vi "Add to Scene.vi"(8 "error in (no error)":errorcluster, 9 "Color":T1={"Red"=0.0, "Green"=0.0, "Blue"=1.0, "Alpha"=1.0}, 10 "Scene Object In":refnum<vi>, 11 "Cube in":refnum<class "Cube.lvclass">) -> (0 "error out":errorcluster, 2 "Scene Object Out":refnum<vi>, 3 "Cube out":refnum<class "Cube.lvclass">)   [LabVIEW 2019, in "22.lvlib" / "Cube.lvclass"]
uses:
  Cube.lvclass
  <vilib>/picture/3D Picture Control/Object/Create Object (drawable).vi
  <vilib>/picture/3D Picture Control/Object/Create Object (name).vi
  <vilib>/picture/3D Picture Control/Object/Add Object (no reference).vi
  <vilib>/picture/3D Picture Control/Object/Add Object (reference).vi
  <vilib>/picture/3D Picture Control/NI_3D Picture Control.lvlib
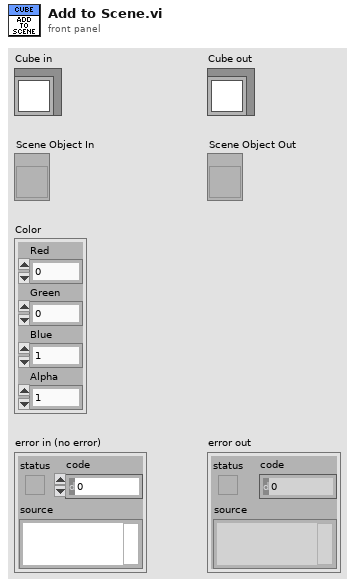
[diagram p1: front panel]
types:
  T1 = cluster{"Red":sgl, "Green":sgl, "Blue":sgl, "Alpha":sgl}
  T2 = cluster{"xmin":i64, "xmax":i64, "ymin":i64, "ymax":i64, "zmin":i64, "zmax":i64}
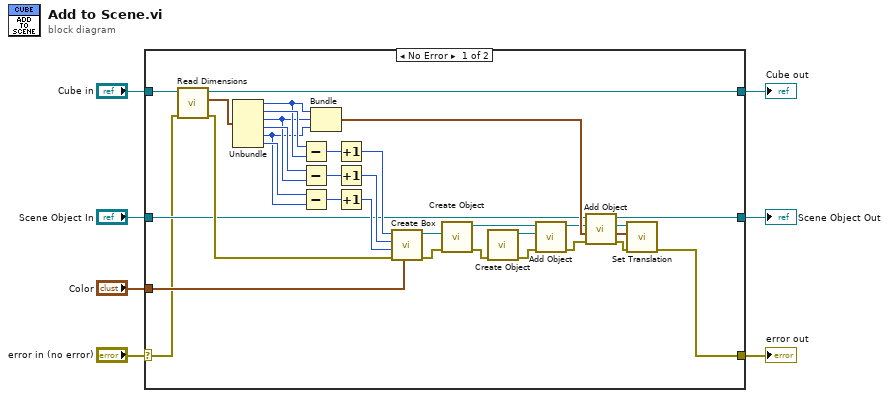
[diagram p0: block diagram]
diagram:
  n1 = case shown="No Error" "error in (no error)" {
    selector: "error in (no error)" -> [w9 w42]
    tunnel: [w13 w42] -> w6
    tunnel: [w39 w41] -> w4
    tunnel: "Cube in" -> [w38 w41]
    tunnel: "Color" -> [w17 _]
    tunnel: "Scene Object In" -> [w15 w40]
    tunnel: [w14 w40] -> w1
    frame No Error {
      n2 = call-dynamic "Read Dimensions.vi"("error in (no error)"=w9, "Cube in"=w38) -> ("error out"=w21:errorcluster, "Dimensions"=w37:T2, "Cube out"=w39:refnum<class "Cube.lvclass">)  [unwired: 7 in]
      n3 = Unbundle(w37) -> ("xmin"=w25:i64, "xmax"=w36:i64, "ymin"=w24:i64, "ymax"=w32:i64, "zmin"=w23:i64, "zmax"=w29:i64)
      n4 = Subtract(x=w36, y=w25) -> (x-y=w35:i64)
      n5 = Subtract(x=w32, y=w24) -> (x-y=w33:i64)
      n6 = Subtract(x=w29, y=w23) -> (x-y=w30:i64)
      n7 = Bundle("xmin"=w25, "ymin"=w24, "zmin"=w23) -> (w22:cluster{"xmin":i64, "ymin":i64, "zmin":i64})  [unwired: 1 in]
      n8 = Increment(x=w35) -> (x+1=w34:i64)
      n9 = Increment(x=w33) -> (x+1=w31:i64)
      n10 = Increment(x=w30) -> (x+1=w28:i64)
      n11 = call <vilib>:"Create Box.vi"("Color"=w17, "error in (no error)"=w21, "Length Z"=w28, "Length Y"=w31, "Length X"=w34) -> ("error out"=w16:errorcluster, "New Box Refnum"=w27:refnum<vi>)  [unwired: 5 in]
      n12 = call-poly <vilib>:"Create Object.vi"("error in (no error)"=w16, "Geometry"=w27) -> ("error out"=w12:errorcluster, "Scene:New Object"=w20:refnum<vi>)  [unwired: 8 in]
      n13 = call-poly <vilib>:"Create Object.vi"("error in (no error)"=w12) -> ("error out"=w11:errorcluster, "Scene:New Object"=w18:refnum<vi>)  [unwired: 9 in]
      n14 = call-poly <vilib>:"Add Object.vi"("error in (no error)"=w11, "New Object In"=w18, "Scene Object In"=w20) -> ("error out"=w10:errorcluster, "Scene Object Out"=w19:refnum<vi>)  [unwired: 7 in]
      n15 = call-poly <vilib>:"Add Object.vi"("error in (no error)"=w10, "New Object In"=w19, "Scene Object In"=w15) -> ("error out"=w8:errorcluster, "New Object Out"=w26:refnum<vi>, "Scene Object Out"=w14:refnum<vi>)  [unwired: 6 in]
      n16 = call <vilib>:"Set Translation.vi"("error in (no error)"=w8, "Translation"=w22, "Scene Object"=w26) -> ("error out"=w13:errorcluster)  [unwired: 7 in, 1 out]
    }
    frame Error {
    }
  }
  "error out" <- w6
  "Cube out" <- w4
  "Scene Object Out" <- w1
